vi "PortCTeleOp.vi"(9 "Robot":T1, 10 "Axes":dbl[](array[numeric]), 11 "Buttons":bool[](array[boolean])) -> ()   [LabVIEW 2015]
uses:
  Robot Type Def.ctl
  Framework/JoystickMappingNamesTypeDef.ctl
  Framework/Robot Global Data.vi
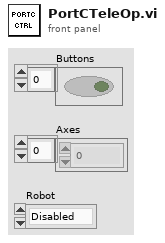
[diagram p1: front panel]
types:
  T1 = typedef "Robot Type Def.ctl" = enum32{"Disabled", "Ghost", "Casper", "Lofty", "Board", "RaceRobot", "Casper 2.0", "Excalibot 2.0"}
  T2 = typedef "JoystickMappingNamesTypeDef.ctl" = enum16{"Shoot Button", "Retrieve Button", "Arm Control", "High Gear", "Low Gear", "Enable PTO", "Disable PTO", "PortC Control", "PortC Up", "PortC Down", "Lift Control", "Drive VBus"}
  T3 = typedef "PortC Settings Type Def.ctl" = cluster{"Down":dbl, "Up":dbl, "Increments":dbl}
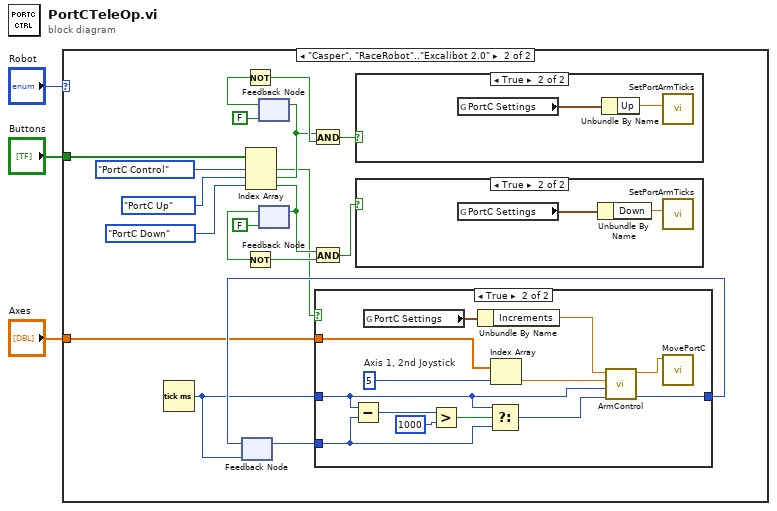
[diagram p0: block diagram]
diagram:
  n1 = case shown="\"Casper\", \"RaceRobot\"..\"Excalibot 2.0\"" "Robot" {
    tunnel: "Buttons" -> [_ w22]
    tunnel: "Axes" -> [_ w6]
    frame "Disabled", Default {
    }
    frame "Casper", "RaceRobot".."Excalibot 2.0" {
      n2 = Tick Count (ms)() -> (millisecond timer value=w4:u32)
      n3 = feedback #1(w4) -> (w7:u32)
      n4 = Index Array(array=w22, index #1=JoystickMappingNamesTypeDef."PortC Control" ("Joystick Button Names"), index #2=JoystickMappingNamesTypeDef."PortC Up" ("Joystick Button Names"), index #3=JoystickMappingNamesTypeDef."PortC Down" ("Joystick Button Names")) -> (element #1=w5:bool, element #2=w15:bool, element #3=w10:bool)
      n5 = feedback #2(FALSE) -> (w18:bool)
      n6 = Not(x=w18) -> (.not. x?=w19:bool)
      n7 = feedback-in #2(w15) -> ()
      n8 = feedback #3(FALSE) -> (w11:bool)
      n9 = Not(x=w11) -> (.not. x?=w12:bool)
      n10 = feedback-in #3(w10) -> ()
      n11 = And(x=w15, y=w19) -> (x .and. y?=w14:bool)
      n12 = And(x=w10, y=w12) -> (x .and. y?=w9:bool)
      n13 = case shown="True" w5 {
        tunnel: w6 -> [_ w35]
        tunnel: [w23 w33] -> w8
        tunnel: w7 -> [_ w29]
        tunnel: w4 -> [w23 w25]
        frame False {
        }
        frame True {
          w36 = 5  # Axis 1, 2nd Joystick
          n14 = Subtract(x=w25, y=w29) -> (x-y=w32:u32)
          n15 = global read "Robot Global Data.vi" "PortC Settings"() -> (w24:T3)
          n16 = Greater?(x=w32, y=u32 1000) -> (0:w30:bool)
          n17 = Unbundle By Name(w24) -> ("Increments"=w27:dbl)
          n18 = Select(t=w25, s=w30, f=w29) -> (s? t:f=w28:u32)
          n19 = Index Array(array=w35, index=w36) -> (element=w34:dbl)
          n20 = call "ArmControl.vi"("Last Increment time"=w28, "Current time"=w25, "Joystick"=w34, "Increment"=w27) -> ("Last Time"=w33:u32, "Increment Amount"=w26:dbl)  [unwired: 6 in]
          n21 = call "MovePortC.vi"("Angle"=w26) -> ()  [unwired: 10 in, 1 out]
        }
      }
      n22 = feedback-in #1(w8) -> ()
      n23 = case shown="True" w14 {
        frame False {
        }
        frame True {
          n24 = global read "Robot Global Data.vi" "PortC Settings"() -> (w40:T3)
          n25 = Unbundle By Name(w40) -> ("Up"=w39:dbl)
          n26 = call "SetPortArmTicks.vi"("Ticks"=w39) -> ()  [unwired: 10 in, 1 out]
        }
      }
      n27 = case shown="True" w9 {
        frame False {
        }
        frame True {
          n28 = global read "Robot Global Data.vi" "PortC Settings"() -> (w38:T3)
          n29 = Unbundle By Name(w38) -> ("Down"=w37:dbl)
          n30 = call "SetPortArmTicks.vi"("Ticks"=w37) -> ()  [unwired: 10 in, 1 out]
        }
      }
    }
  }
